vi "Unreserve.vi"(0 "object in":refnum<class "HPS-17000-PowerModule.lvclass">, 11 "Error In":errorcluster) -> (4 "object out":refnum<class "HPS-17000-PowerModule.lvclass">, 15 "Error Out":errorcluster)   [LabVIEW 2023, in "HPS-17000-PowerModule.lvlib" / "HPS-17000-PowerModule.lvclass"]
uses:
  HPS-17000-PowerModule.lvclass
  <instrlib>/HPS-17000/Internal/Unreserve Multi.vi
  <instrlib>/HPS-17000/HPS-17000.lvclass
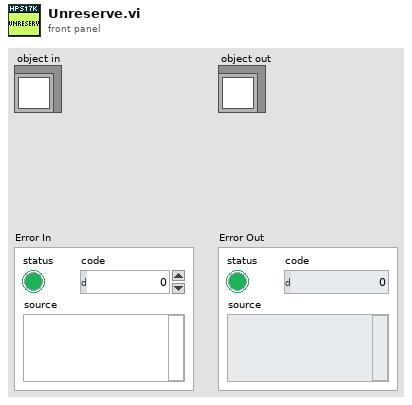
[diagram p1: front panel]
types:
  T1 = typedef "HPS-17000-PowerModule.lvlib/HPS-17000-PowerModule.lvclass/ObjectAttributes.ctl" = cluster{"HPS17000 IP Addresses":string[], "HPS Topology":enum16{"SINGLE", "MULTI"}, "GM ID":string, "TSN NIC IP Address":string, "HPS17000 Refs":refnum<class "HPS-17000.lvclass">[], "Stream Queues":refnum<queue>[], "connected":bool, "reserved":bool, "events":T2, "nibatterycycler_grpc_Setpoint":T3, "last timestamp":i64, "setpoint stream config":T4, "mode":T5, "range":T6}
  T2 = typedef "HPS-17000.lvclass/Multi-Cycler Events.ctl" = cluster{"heartbeats events":refnum<user-event>[], "faults events":refnum<user-event>[], "network sync event":refnum<user-event>[], "setpoint status event":refnum<user-event>[]}
  T3 = typedef "NI_BC_client.lvlib/nibatterycycler_grpc_Setpoint.ctl" = cluster{"voltage":sgl, "current":sgl, "min_power":sgl, "max_power":sgl, "resistance":sgl}
  T4 = typedef "Cycler.lvclass/Setpoint Stream Basic Config.ctl" = cluster{"local address":string, "receiver port":u16}
  T5 = typedef "HPS-17000-PowerModule.lvlib/HPS-17000-PowerModule.lvclass/Mode.ctl" = u16
  T6 = typedef "PowerModuleInterface.lvlibp/PowerModuleInterface.lvclass/Range.ctl" = cluster{"Current Max (A)":dbl, "Current Min (A)":dbl, "Voltage Max (V)":dbl, "Voltage Min (V)":dbl}
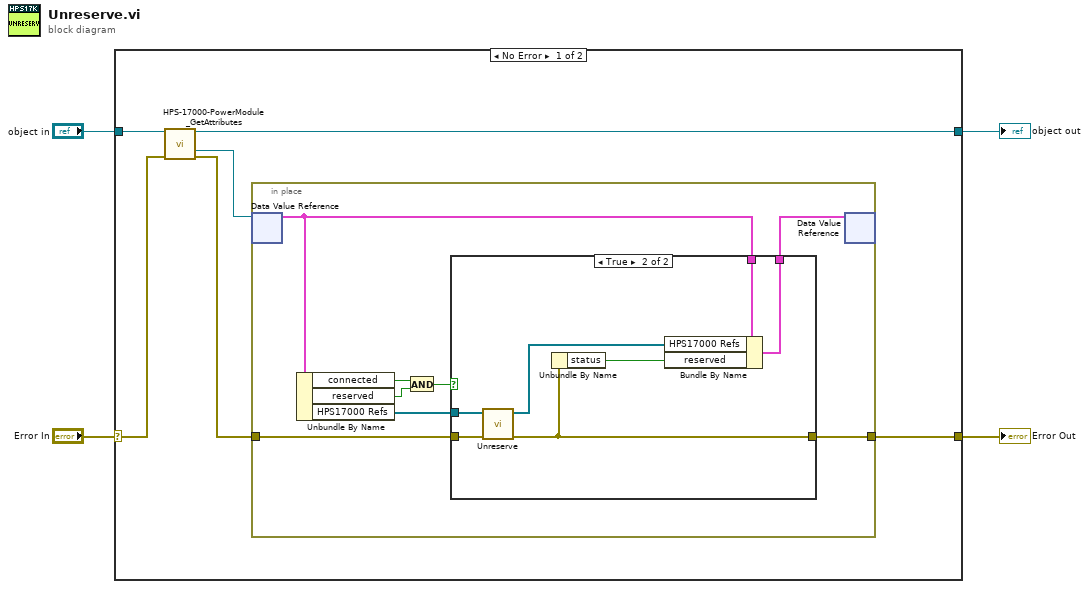
[diagram p0: block diagram]
diagram:
  n1 = case shown="No Error" "Error In" {
    selector: "Error In" -> [w9 w28]
    tunnel: "object in" -> [w10 w29]
    tunnel: [w5 w29] -> w2
    tunnel: [w6 w28] -> w3
    frame No Error {
      n2 = call "HPS-17000-PowerModule_GetAttributes.vi"("reference in"=w10, "Error In"=w9) -> ("reference out"=w5:refnum<class "HPS-17000-PowerModule.lvclass">, "DataRef"=w8:refnum<data-value>, "Error Out"=w7:errorcluster)  [unwired: 10 in, 1 out]
      n3 = in-place {
        in-place-border: w7 -> [w16]
        in-place-border: [w15] -> w6
        n4 = in-place-dvr #1(w8) -> (w17:T1)  [unwired: 1 out]
        n5 = Unbundle By Name(w17) -> ("connected"=w13:bool, "reserved"=w12:bool, "HPS17000 Refs"=w14:refnum<class "HPS-17000.lvclass">[])
        n6 = And(x=w13, y=w12) -> (x .and. y?=w11:bool)
        n7 = case shown="True" w11 {
          tunnel: [w20 w27] -> w18
          tunnel: w17 -> [w20 w26]
          tunnel: w16 -> [w19 w24]
          tunnel: [w19 w22] -> w15
          tunnel: w14 -> [_ w25]
          frame False {
          }
          frame True {
            n8 = call-poly <instrlib>:"Unreserve.vi"("error in"=w24, "cycler refs in"=w25) -> ("error out"=w22:errorcluster, "cycler refs out"=w23:refnum<class "HPS-17000.lvclass">[])  [unwired: 8 in]
            n9 = Unbundle By Name(w22) -> ("status"=w21:bool)
            n10 = Bundle By Name(cluster=w26, "HPS17000 Refs"=w23, "reserved"=w21) -> (w27:T1)
          }
        }
        n11 = in-place-dvr #1(w18) -> ()  [unwired: 2 out]
      }
    }
    frame Error {
    }
  }
  "Error Out" <- w3
  "object out" <- w2
